vi "Build.vi"(8 "error in (no error)":errorcluster, 10 "collect dependencies? (F)":bool, 11 "SDIST in":refnum<class "NI_AB_API_SDIST.lvclass">) -> (0 "error out":errorcluster, 1 "Dependencies":T1[](array[typedef]), 2 "GeneratedFiles":path[](array[path]), 3 "SDIST out":refnum<class "NI_AB_API_SDIST.lvclass">)   [LabVIEW 2020, in "NI_AB_API_SDIST.lvclass"]
uses:
  <vilib>/AppBuilder/AB_API/SDIST/NI_AB_API_SDIST.lvclass
  <vilib>/AppBuilder/AB_Dependency.ctl
  <vilib>/Utility/lvfile.llb/LVFileType.ctl
  <vilib>/AppBuilder/AB_API/Build/NI_AB_API_Build.lvclass
  <vilib>/Utility/lvfile.llb/NI_FileType.lvlib
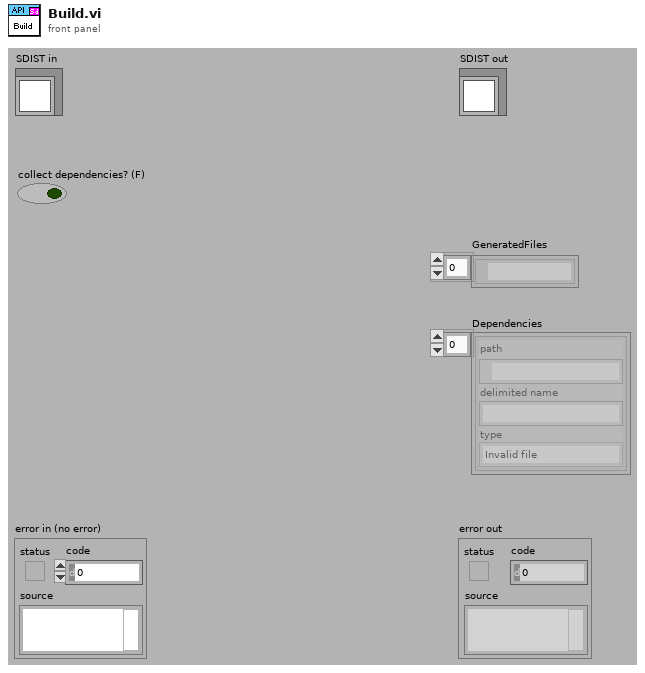
[diagram p1: front panel]
types:
  T1 = typedef "AB_Dependency.ctl" = cluster{"path":path, "delimited name":string, "type":T2}
  T2 = typedef "NI_FileType.lvlib/LVFileType.ctl" = enum32{"Invalid file", "Unknown type", "Instrument", "Control", "Polymorphic VI", "Project", "Library", "LVClass", "XControl", "XNode", "Shared library", ".NET assembly", "ActiveX interface", "CIN", "Run-time menu", "Palette menu", "Help file", "LLB", "XNode Edit Dependency", "Class Private Data Control", "Statechart", "MathScript .m file", "Ladder Diagram", "LVLibp", "XNode Build Dependency"}
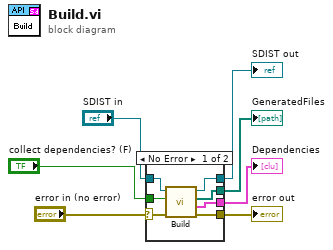
[diagram p0: block diagram]
diagram:
  n1 = case shown="No Error" "error in (no error)" {
    selector: "error in (no error)" -> [w10 w16]
    tunnel: [w11 w16] -> w6
    tunnel: [w13 w15] -> w4
    tunnel: "SDIST in" -> [w14 w15]
    tunnel: [w12 _] -> w3
    tunnel: [w9 _] -> w2
    tunnel: "collect dependencies? (F)" -> [w8 _]
    frame No Error {
      n2 = call-parent "Build.vi"("error in (no error)"=w10, "collect dependencies? (F)"=w8, "Build in"=w14) -> ("error out"=w11:errorcluster, "Dependencies"=w9:T1[], "GeneratedFiles"=w12:path[], "Build out"=w13:refnum<class "NI_AB_API_SDIST.lvclass">)  [unwired: 5 in]
    }
    frame Error {
    }
  }
  "error out" <- w6
  "SDIST out" <- w4
  "GeneratedFiles" <- w3
  "Dependencies" <- w2
